vi "Configure Control Mode.vi"(8 "error in (no error)":errorcluster, 9 "Control Mode (0: BUS/RS232)":T1(ring), 10 "Node (3)":u8=3 caption="Node" min=3 max=128 step=1, 11 "VISA resource name":refnum<visa-resource-name>) -> (0 "error out":errorcluster, 3 "VISA resource name out":refnum<visa-resource-name>)   [LabVIEW 2024, in "Bronkhorst FLOW-BUS.lvlib"]
doc: "Configures the control mode of the instrument. The control mode is used for switching between different functions of a digital meter or controller. Several modes are available."
uses:
  Bronkhorst FLOW-BUS.lvlib
  Private/FLOW-BUS RW.ctl
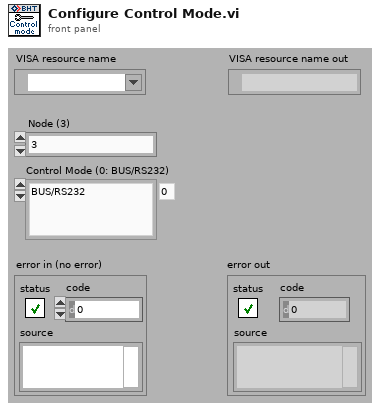
[diagram p1: front panel]
types:
  T1 = enum32{"BUS/RS232", "Analog input", "FLOW-BUS slave", "Valve close", "Controller idle", "Testing mode", "Tuning mode", "Setpoint 100%", "Valve fully open", "Calibration mode", "Analog slave", "Keyboard or FLOW-BUS setpoint", "Setpoint 0%", "FLOW-BUS analog slave", "(FPP) Range select mode", "(FPP) Manual start sensor select, automatic end sensor", "(FPP) Automatic start sensor select, manual end sensor", "(FPP) Automatic start and end sensor", "RS232 Setpoint", "RS232 broadcast mode", "Valve stearing (valve = setpoint)", "Analog valve stearing (valve = analog setpoint)", "Valve safe state"}
  T2 = typedef "Bronkhorst FLOW-BUS.lvlib/FLOW-BUS RW.ctl" = cluster{"Node Address (3)":u8, "Communication Command":enum16{"Status message", "Send parameter with destination address and 00 response", "Send parameter with destination address", "Request parameter"}, "Process (0)":u16, "Parameter (0)":u16, "Data Type (0: Character)":enum16{"Character", "Integer", "Float or Long", "String"}, "Data for Char, Int, or Long (0)":u32, "Data for Float (0)":sgl, "Data for String":string, "Length of Requested String (0)":u8}
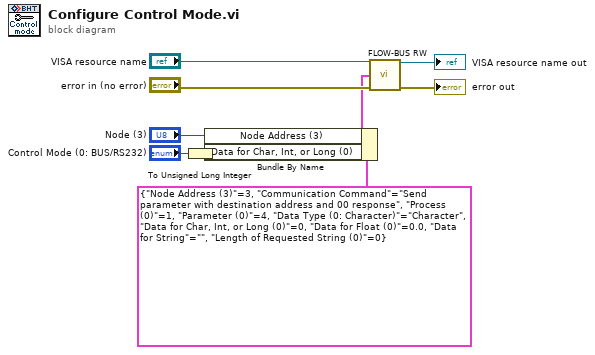
[diagram p0: block diagram]
diagram:
  n1 = To Unsigned Long Integer(number="Control Mode (0: BUS/RS232)") -> (unsigned 32bit integer=w1:u32)
  n2 = Bundle By Name(cluster=T2 {"Node Address (3)"=3, "Communication Command"=enum."Send parameter with destination address and 00 response", "Process (0)"=1, "Parameter (0)"=4, "Data Type (0: Character)"=enum."Character", "Data for Char, Int, or Long (0)"=0, "Data for Float (0)"=0.0, "Data for String"="", "Length of Requested String (0)"=0} ("FLOW-BUS Command Settings"), "Node Address (3)"="Node (3)", "Data for Char, Int, or Long (0)"=w1) -> (w4:T2)
  n3 = call "FLOW-BUS RW.vi"("VISA resource name"="VISA resource name", "FLOW-BUS Command Settings"=w4, "error in (no error)"="error in (no error)") -> ("VISA resource name out"=→"VISA resource name out":refnum<visa-resource-name>, "error out"=→"error out":errorcluster)  [unwired: 8 in, 3 out]
